vi "Autonomous Independent.vi"() -> ()   [LabVIEW 2015]
doc: "This VI is called when autonomous begins, and will automatically be terminated when autonomous ends. You can carry out timed or sensor driven robot movement independently without needing to return to the caller."
uses:
  Controls/Time.ctl
  Controls/Speed.ctl
  <vilib>/Rock Robotics/WPI/Solenoid/WPI_SolenoidValue.ctl
  <vilib>/Rock Robotics/Network Tables/NT Read String.vi
  <vilib>/Rock Robotics/WPI/Utilities/WPI_GetSetVariantRefNum.vi
  <vilib>/Rock Robotics/Network Tables/NT Write Numeric Array.vi
  <vilib>/Rock Robotics/WPI/Solenoid/WPI_SolenoidSetEnum.vi
  <vilib>/Rock Robotics/Network Tables/NT Write Boolean.vi
  <vilib>/Rock Robotics/Network Tables/NT Read Boolean.vi
panel:
  out "Green":bool
  # "Be sure to right-click and choose Data Operations>>Make Current Value default if you want to save the array values with the VI"
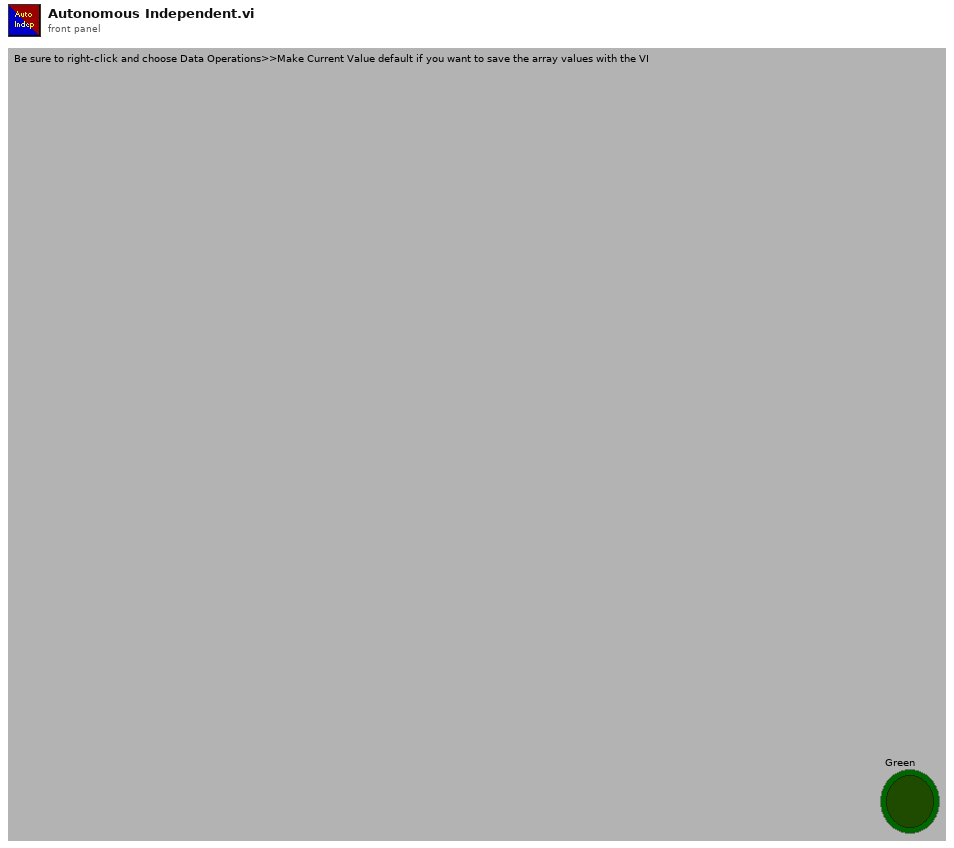
[diagram p1: front panel]
types:
  T1 = typedef "WPI_MotorControlDeviceRef.ctl" = cluster{"DeviceStatus":errorcluster, "Type":T2, "PWM":cluster{"PWM Channel":T3, "DeadBand":T4}, "CAN":cluster{"Device Number":u8, "Control Mode":T5, "Semaphore":T6, "Max Vout":dbl, "TalonSRX Control Mode":T7}, "Invert":bool}
  T2 = typedef "WPI_MotorControlType.ctl" = enum16{"PWM", "CAN", "CANTalonSRX"}
  T3 = typedef "FPGA_DIOPWMChannel.ctl" = enum8{"PWM 0", "PWM 1", "PWM 2", "PWM 3", "PWM 4", "PWM 5", "PWM 6", "PWM 7", "PWM 8", "PWM 9", "PWM MXP 0", "PWM MXP 1", "PWM MXP 2", "PWM MXP 3", "PWM MXP 4", "PWM MXP 5", "PWM MXP 6", "PWM MXP 7", "PWM MXP 8", "PWM MXP 9", "Invalid"}
  T4 = typedef "WPI_PWMDeadband.ctl" = cluster{"Name":string, "maxPositivePwm":i32, "minPositivePwm":i32, "centerPwm":i32, "maxNegativePwm":i32, "minNegativePwm":i32, "angularRange":u16}
  T5 = typedef "WPI_CANJaguar_ControlMode.ctl" = enum8{"Percent VBus", "Current", "Speed", "Position", "Voltage"}
  T6 = typedef "Semaphore RefNum" = refnum<k1>
  T7 = typedef "WPI_CANTalonSRX_APIControlMode.ctl" = enum8{"Percent VBus", "Speed", "Position", "Slave", "Unchanged / Invalid", "Voltage Compensation", "Current", "Motion Profile"}
  T8 = typedef "WPI_JoystickDevRef.ctl" = cluster{"Device":T9}
  T9 = typedef "WPI_JoystickDeviceEnum.ctl" = enum16{"USB 0", "USB 1", "USB 2", "USB 3", "USB 4", "USB 5"}
  T10 = typedef "WPI_RobotDriveDevRef.ctl" = cluster{"DevStatus":errorcluster, "Motors[]":T1[], "Square Inputs":bool, "Max Output":dbl}
  T11 = typedef "Speed.ctl" = dbl
  T12 = typedef "Time.ctl" = dbl
  T13 = typedef "WPI_SolenoidValue.ctl" = enum16{"Off", "On", "Forward", "Reverse"}
  T14 = typedef "WPI_SolenoidDevRef.ctl" = cluster{"DevStatus":errorcluster, "Pneumatics Control Module":u8, "Forward Solenoid Channel":T15, "Reverse Solenoid Channel":T15}
  T15 = typedef "WPI_SolenoidChannel.ctl" = enum8{"Solenoid 0", "Solenoid 1", "Solenoid 2", "Solenoid 3", "Solenoid 4", "Solenoid 5", "Solenoid 6", "Solenoid 7", "Invalid"}
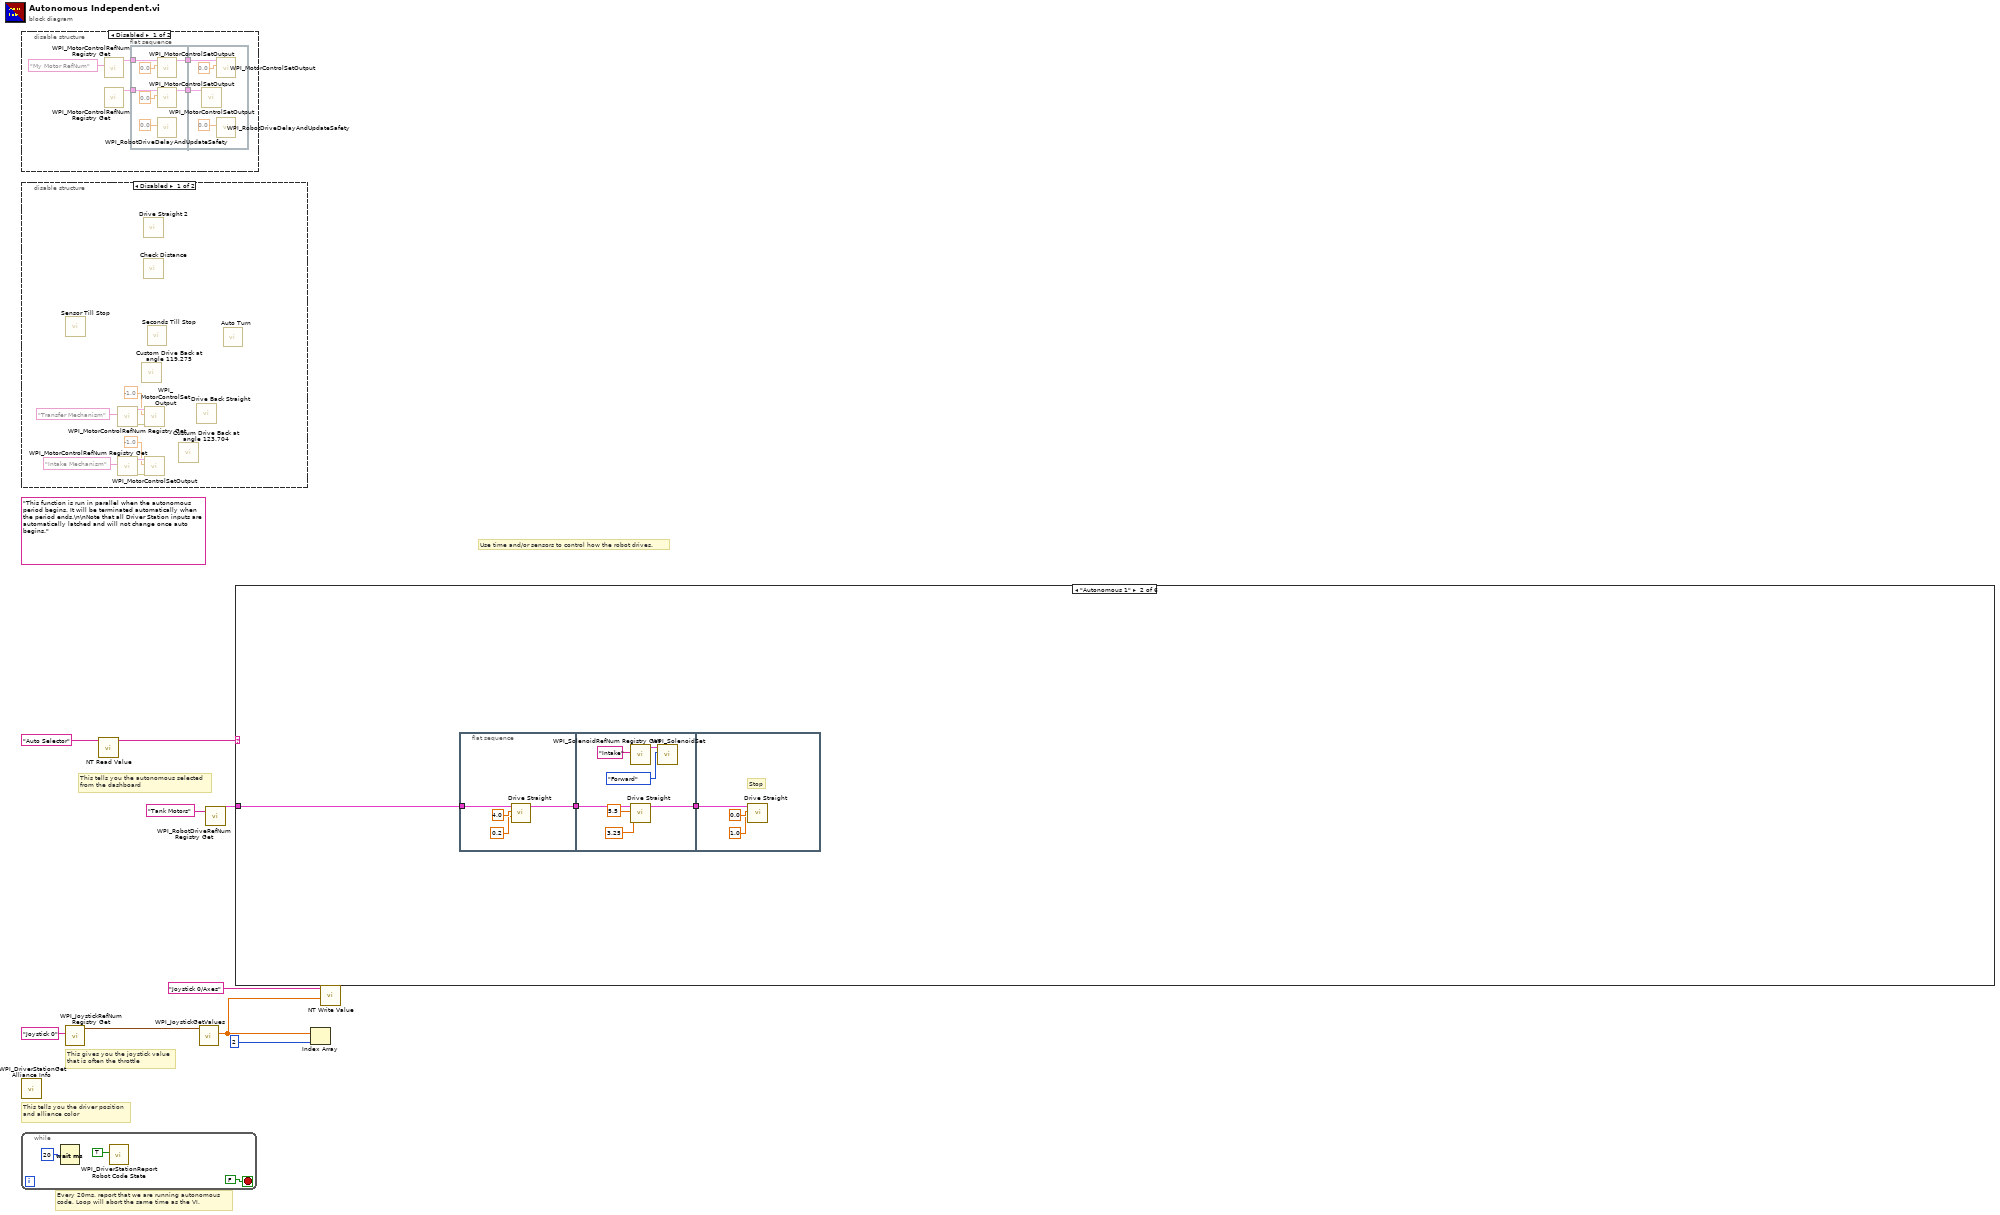
[diagram p0: block diagram]
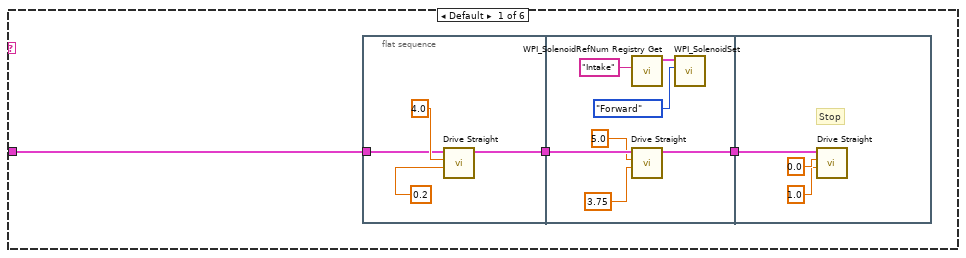
[diagram p4: hidden frame]
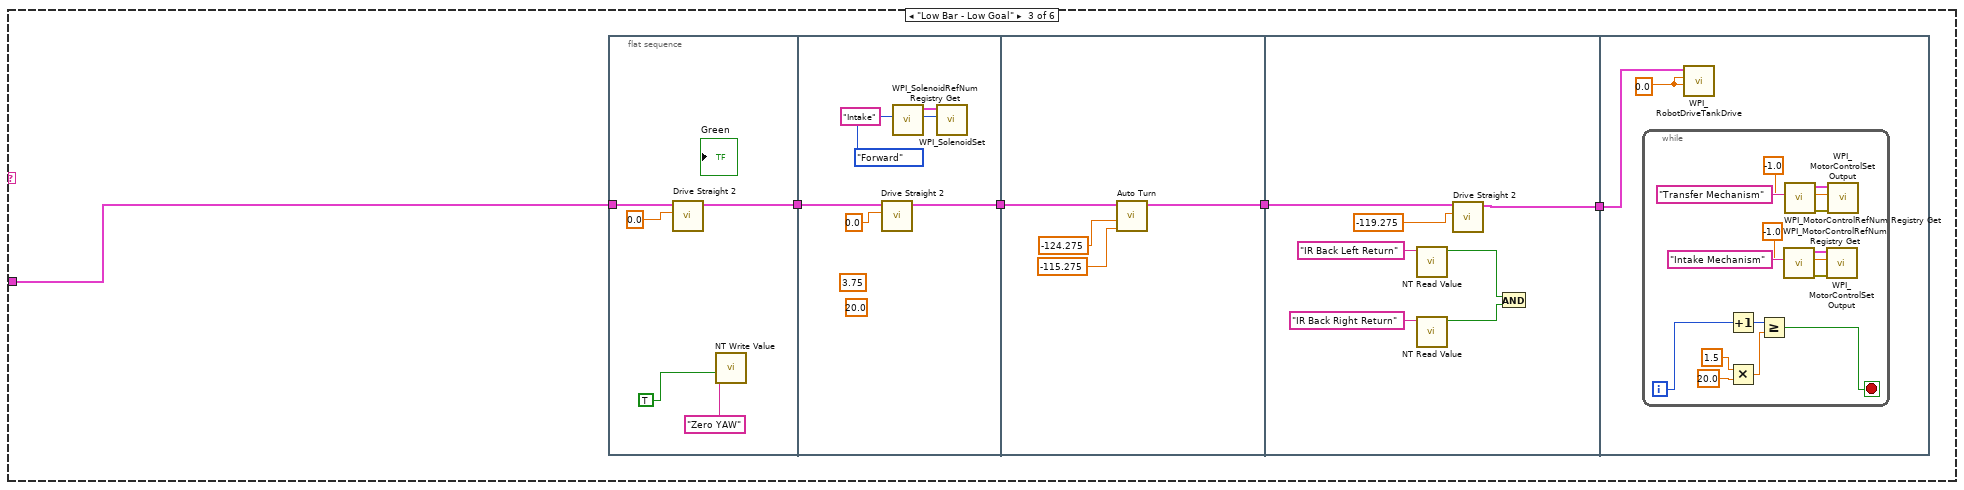
[diagram p5: hidden frame]
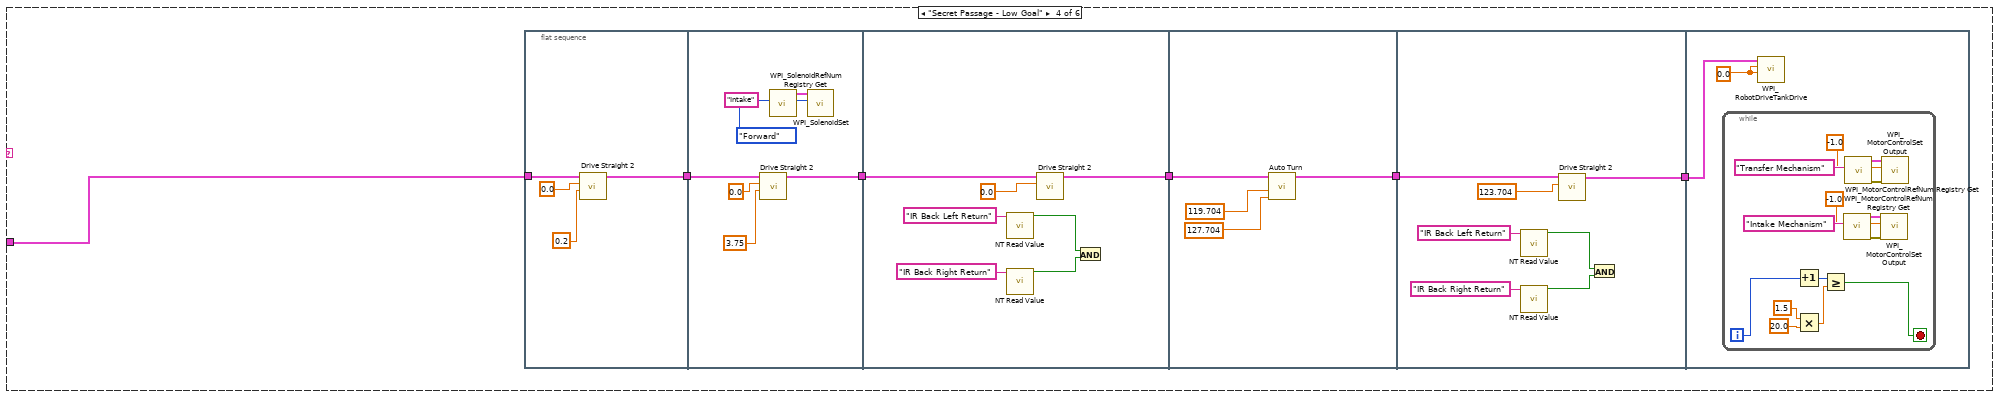
[diagram p6: hidden frame]
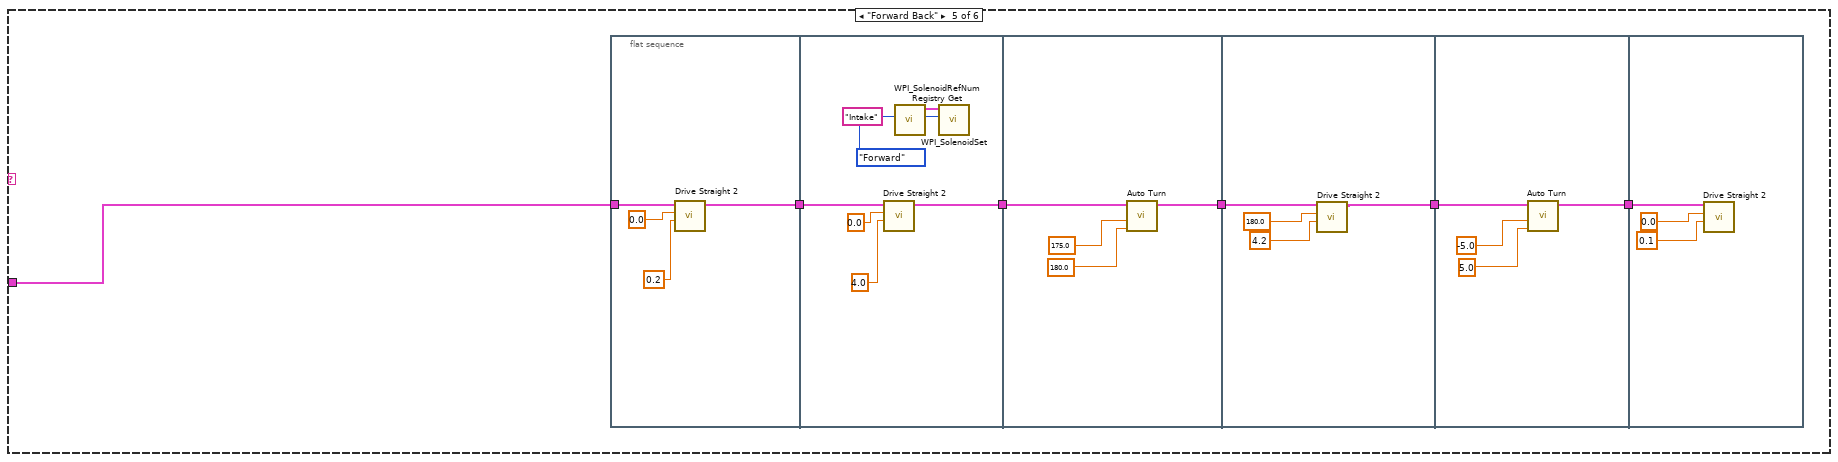
[diagram p7: hidden frame]
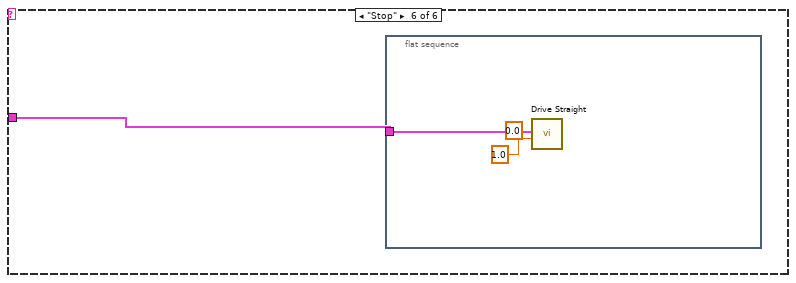
[diagram p8: hidden frame]
diagram:
  (unwired) "This function is run in parallel when the autonomous period begins. It will be terminated automatically when the period ends.\n\nNote that all Driver Station inputs are automatically latched and will not change once auto begins."
  # "This gives you the joystick value\nthat is often the throttle"
  # "This tells you the autonomous selected\nfrom the dashboard"
  # "Every 20ms, report that we are running autonomous\ncode. Loop will abort the same time as the VI."
  # "Use time and/or sensors to control how the robot drives."
  # "This tells you the driver position\nand alliance color"
  n1 = disable-structure shown="Disabled" {
    frame Disabled {
      n2 = call <vilib>:"WPI_MotorControlRefNum Registry Get.vi"("refnum name"="My Motor RefNum") -> ("MotorControlDevRef"=w11:T1)  [unwired: 9 in, 1 out]
      n3 = call <vilib>:"WPI_MotorControlRefNum Registry Get.vi"() -> ("MotorControlDevRef"=w10:T1)  [unwired: 10 in, 1 out]
      n4 = flat-sequence {
        tunnel: w11 -> [w21]
        tunnel: [w18] -> w14
        tunnel: w10 -> [w15]
        tunnel: [w16] -> w13
        tunnel: w14 -> [w23]
        tunnel: w13 -> [w22]
        frame #0 {
          n5 = call <vilib>:"WPI_MotorControlSetOutput.vi"("Output"=0.0, "MotorControlDevRef"=w21) -> ("MotorControlDevRef"=w18:T1)  [unwired: 7 in, 2 out]
          n6 = call <vilib>:"WPI_MotorControlSetOutput.vi"("Output"=0.0, "MotorControlDevRef"=w15) -> ("MotorControlDevRef"=w16:T1)  [unwired: 7 in, 2 out]
          n7 = call <vilib>:"WPI_RobotDriveDelayAndUpdateSafety.vi"("Delay (s)"=0.0) -> ()  [unwired: 9 in, 2 out]
        }
        frame #1 {
          n8 = call <vilib>:"WPI_MotorControlSetOutput.vi"("MotorControlDevRef"=w22) -> ()  [unwired: 8 in, 3 out]
          n9 = call <vilib>:"WPI_MotorControlSetOutput.vi"("Output"=0.0, "MotorControlDevRef"=w23) -> ()  [unwired: 7 in, 3 out]
          n10 = call <vilib>:"WPI_RobotDriveDelayAndUpdateSafety.vi"("Delay (s)"=0.0) -> ()  [unwired: 9 in, 2 out]
        }
      }
    }
    frame Enabled {
    }
  }
  n11 = disable-structure shown="Disabled" {
    frame Disabled {
      n12 = call "Sensor Till Stop.vi"() -> ()  [unwired: 11 in, 1 out]
      n13 = call <vilib>:"WPI_MotorControlRefNum Registry Get.vi"("refnum name"="Transfer Mechanism") -> ("error out"=w30:errorcluster, "MotorControlDevRef"=w28:T1)  [unwired: 9 in]
      n14 = call <vilib>:"WPI_MotorControlRefNum Registry Get.vi"("refnum name"="Intake Mechanism") -> ("error out"=w33:errorcluster, "MotorControlDevRef"=w32:T1)  [unwired: 9 in]
      n15 = call "Custom Drive Back at angle 119.275.vi"() -> ()  [unwired: 10 in, 2 out]
      n16 = call "Drive Straight 2.vi"() -> ()  [unwired: 11 in, 1 out]
      n17 = call "Check Distance.vi"() -> ()  [unwired: 11 in, 1 out]
      n18 = call <vilib>:"WPI_MotorControlSetOutput.vi"("error in (no error)"=w30, "Output"=-1.0, "MotorControlDevRef"=w28) -> ()  [unwired: 6 in, 3 out]
      n19 = call <vilib>:"WPI_MotorControlSetOutput.vi"("error in (no error)"=w33, "Output"=-1.0, "MotorControlDevRef"=w32) -> ()  [unwired: 6 in, 3 out]
      n20 = call "Seconds Till Stop.vi"() -> ()  [unwired: 11 in, 1 out]
      n21 = call "Custum Drive Back at angle 123.704.vi"() -> ()  [unwired: 10 in, 2 out]
      n22 = call "Drive Back Straight.vi"() -> ()  [unwired: 10 in, 2 out]
      n23 = call "Auto Turn.vi"() -> ()  [unwired: 11 in, 1 out]
    }
    frame Enabled {
    }
  }
  n24 = call <vilib>:"WPI_DriverStationGet Alliance Info.vi"() -> ()  [unwired: 12 out]
  n25 = while {
    stop <- FALSE stop-if-true
    n26 = Wait (ms)(milliseconds to wait=u32 20) -> ()  [unwired: 1 out]
    n27 = call <vilib>:"WPI_DriverStationReport Robot Code State.vi"("Autonomous"=TRUE) -> ()  [unwired: 10 in, 1 out]
  }
  n28 = call <vilib>:"WPI_JoystickRefNum Registry Get.vi"("refnum name"="Joystick 0") -> ("JoystickDevRef"=w6:T8)  [unwired: 1 in, 9 out]
  n29 = call-poly <vilib>:"NT Read Value.vi"("Name"="Auto Selector") -> ("String"=w8:string)  [unwired: 9 in, 1 out]
  n30 = call <vilib>:"WPI_JoystickGetValues.vi"("JoystickDevRef"=w6) -> ("Axes"=w4:dbl[])  [unwired: 6 in, 4 out]
  n31 = call <vilib>:"WPI_RobotDriveRefNum Registry Get.vi"("refnum name"="Tank Motors") -> ("RobotDriveDevRef"=w1:T10)  [unwired: 9 in, 1 out]
  n32 = case shown="\"Autonomous 1\"" w8 {
    tunnel: w1 -> [w37 w54 w75 w119 w170 w197]
    frame Default {
      n33 = flat-sequence {
        tunnel: [w41] -> w39
        tunnel: w37 -> [w40]
        tunnel: w39 -> [w47]
        tunnel: [w44] -> w38
        tunnel: w38 -> [w53]
        frame #0 {
          n34 = call "Drive Straight.vi"("Time"=T12 0.2, "Speed"=T11 4.0, "RobotDriveDevRef"=w40) -> ("RobotDriveDevRef 2"=w41:T10)  [unwired: 8 in]
        }
        frame #1 {
          n35 = call <vilib>:"WPI_SolenoidRefNum Registry Get.vi"("refnum name"="Intake") -> ("SolenoidDevRef"=w49:T14)  [unwired: 9 in, 1 out]
          n36 = call "Drive Straight.vi"("Time"=T12 3.75, "Speed"=T11 5.0, "RobotDriveDevRef"=w47) -> ("RobotDriveDevRef 2"=w44:T10)  [unwired: 8 in]
          n37 = call-poly <vilib>:"WPI_SolenoidSet.vi"("Value"=WPI_SolenoidValue."Forward", "SolenoidDevRef"=w49) -> ()  [unwired: 1 in, 9 out]
        }
        frame #2 {
          # "Stop"
          n38 = call "Drive Straight.vi"("Time"=T12 1.0, "Speed"=T11 0.0, "RobotDriveDevRef"=w53) -> ()  [unwired: 8 in, 1 out]
        }
      }
    }
    frame "Autonomous 1" {
      n39 = flat-sequence {
        tunnel: [w58] -> w56
        tunnel: w54 -> [w57]
        tunnel: w56 -> [w67]
        tunnel: [w65] -> w55
        tunnel: w55 -> [w70]
        frame #0 {
          n40 = call "Drive Straight.vi"("Time"=T12 0.2, "Speed"=T11 4.0, "RobotDriveDevRef"=w57) -> ("RobotDriveDevRef 2"=w58:T10)  [unwired: 8 in]
        }
        frame #1 {
          n41 = call <vilib>:"WPI_SolenoidRefNum Registry Get.vi"("refnum name"="Intake") -> ("SolenoidDevRef"=w63:T14)  [unwired: 9 in, 1 out]
          n42 = call "Drive Straight.vi"("Time"=T12 3.25, "Speed"=T11 5.5, "RobotDriveDevRef"=w67) -> ("RobotDriveDevRef 2"=w65:T10)  [unwired: 8 in]
          n43 = call-poly <vilib>:"WPI_SolenoidSet.vi"("Value"=WPI_SolenoidValue."Forward", "SolenoidDevRef"=w63) -> ()  [unwired: 1 in, 9 out]
        }
        frame #2 {
          # "Stop"
          n44 = call "Drive Straight.vi"("Time"=T12 1.0, "Speed"=T11 0.0, "RobotDriveDevRef"=w70) -> ()  [unwired: 8 in, 1 out]
        }
      }
    }
    frame "Low Bar - Low Goal" {
      n45 = flat-sequence {
        tunnel: [w78] -> w73
        tunnel: w75 -> [w80]
        tunnel: w73 -> [w82]
        tunnel: [w81] -> w71
        tunnel: [w90] -> w74
        tunnel: w71 -> [w87]
        tunnel: w74 -> [w92]
        tunnel: [w91] -> w72
        tunnel: w72 -> [w99]
        frame #0 {
          n46 = call "Drive Straight 2.vi"("Angle"=0.0, "RobotDriveDevRef in"=w80) -> ("RobotDriveDevRef out"=w78:T10)  [unwired: 9 in]
          n47 = call-poly <vilib>:"NT Write Value.vi"("Boolean"=TRUE, "Name"="Zero YAW") -> ()  [unwired: 9 in, 1 out]
        }
        frame #1 {
          (unwired) 20.0 ("y")
          (unwired) 3.75 ("Time")
          n48 = call "Drive Straight 2.vi"("Angle"=0.0, "RobotDriveDevRef in"=w82) -> ("RobotDriveDevRef out"=w81:T10)  [unwired: 9 in]
          n49 = call <vilib>:"WPI_SolenoidRefNum Registry Get.vi"("refnum name"="Intake") -> ("SolenoidDevRef"=w85:T14)  [unwired: 9 in, 1 out]
          n50 = call-poly <vilib>:"WPI_SolenoidSet.vi"("Value"=WPI_SolenoidValue."Forward", "SolenoidDevRef"=w85) -> ()  [unwired: 1 in, 9 out]
        }
        frame #2 {
          n51 = call "Auto Turn.vi"("upper limit"=-115.275 ("lower limit"), "lower limit"=-124.275 ("upper limit"), "RobotDriveDevRef"=w87) -> ("RobotDriveDevRef out"=w90:T10)  [unwired: 8 in]
        }
        frame #3 {
          n52 = call-poly <vilib>:"NT Read Value.vi"("Name"="IR Back Left Return") -> ("Boolean"=w94:bool)  [unwired: 9 in, 1 out]
          n53 = call-poly <vilib>:"NT Read Value.vi"("Name"="IR Back Right Return") -> ("Boolean"=w95:bool)  [unwired: 9 in, 1 out]
          n54 = call "Drive Straight 2.vi"("Angle"=-119.275, "RobotDriveDevRef in"=w92) -> ("RobotDriveDevRef out"=w91:T10)  [unwired: 9 in]
          n55 = And(x=w94, y=w95) -> ()  [unwired: 1 out]
        }
        frame #4 {
          w98 = 0.0 ("Angle")
          n56 = while {
            i -> [w101]
            stop <- w100 stop-if-true
            n57 = Increment(x=w101) -> (x+1=w103:i32)
            n58 = Multiply(x=1.5 ("Time"), y=20.0) -> (x*y=w104:dbl)
            n59 = Greater Or Equal?(x=w103, y=w104) -> (x >= y?=w100:bool)
            n60 = call <vilib>:"WPI_MotorControlRefNum Registry Get.vi"("refnum name"="Intake Mechanism") -> ("error out"=w113:errorcluster, "MotorControlDevRef"=w112:T1)  [unwired: 9 in]
            n61 = call <vilib>:"WPI_MotorControlRefNum Registry Get.vi"("refnum name"="Transfer Mechanism") -> ("error out"=w110:errorcluster, "MotorControlDevRef"=w108:T1)  [unwired: 9 in]
            n62 = call <vilib>:"WPI_MotorControlSetOutput.vi"("error in (no error)"=w113, "Output"=-1.0, "MotorControlDevRef"=w112) -> ()  [unwired: 6 in, 3 out]
            n63 = call <vilib>:"WPI_MotorControlSetOutput.vi"("error in (no error)"=w110, "Output"=-1.0, "MotorControlDevRef"=w108) -> ()  [unwired: 6 in, 3 out]
          }
          n64 = call <vilib>:"WPI_RobotDriveTankDrive.vi"("Right axis value"=w98, "Left axis value"=w98, "RobotDriveDevRef"=w99) -> ()  [unwired: 6 in, 3 out]
        }
      }
    }
    frame "Secret Passage - Low Goal" {
      n65 = flat-sequence {
        tunnel: [w121] -> w115
        tunnel: w119 -> [w123]
        tunnel: [w127] -> w118
        tunnel: w115 -> [w125]
        tunnel: w118 -> [w137]
        tunnel: [w135] -> w117
        tunnel: w117 -> [w141]
        tunnel: [w140] -> w116
        tunnel: w116 -> [w143]
        tunnel: [w142] -> w114
        tunnel: w114 -> [w150]
        frame #0 {
          n66 = call "Drive Straight 2.vi"("Time"=0.2, "Angle"=0.0, "RobotDriveDevRef in"=w123) -> ("RobotDriveDevRef out"=w121:T10)  [unwired: 8 in]
        }
        frame #1 {
          n67 = call "Drive Straight 2.vi"("Time"=3.75, "Angle"=0.0, "RobotDriveDevRef in"=w125) -> ("RobotDriveDevRef out"=w127:T10)  [unwired: 8 in]
          n68 = call <vilib>:"WPI_SolenoidRefNum Registry Get.vi"("refnum name"="Intake") -> ("SolenoidDevRef"=w129:T14)  [unwired: 9 in, 1 out]
          n69 = call-poly <vilib>:"WPI_SolenoidSet.vi"("Value"=WPI_SolenoidValue."Forward", "SolenoidDevRef"=w129) -> ()  [unwired: 1 in, 9 out]
        }
        frame #2 {
          n70 = call-poly <vilib>:"NT Read Value.vi"("Name"="IR Back Left Return") -> ("Boolean"=w134:bool)  [unwired: 9 in, 1 out]
          n71 = call-poly <vilib>:"NT Read Value.vi"("Name"="IR Back Right Return") -> ("Boolean"=w133:bool)  [unwired: 9 in, 1 out]
          n72 = call "Drive Straight 2.vi"("Angle"=0.0, "RobotDriveDevRef in"=w137) -> ("RobotDriveDevRef out"=w135:T10)  [unwired: 9 in]
          n73 = And(x=w134, y=w133) -> ()  [unwired: 1 out]
        }
        frame #3 {
          n74 = call "Auto Turn.vi"("upper limit"=127.704, "lower limit"=119.704, "RobotDriveDevRef"=w141) -> ("RobotDriveDevRef out"=w140:T10)  [unwired: 8 in]
        }
        frame #4 {
          n75 = call-poly <vilib>:"NT Read Value.vi"("Name"="IR Back Left Return") -> ("Boolean"=w145:bool)  [unwired: 9 in, 1 out]
          n76 = call-poly <vilib>:"NT Read Value.vi"("Name"="IR Back Right Return") -> ("Boolean"=w146:bool)  [unwired: 9 in, 1 out]
          n77 = call "Drive Straight 2.vi"("Angle"=123.704, "RobotDriveDevRef in"=w143) -> ("RobotDriveDevRef out"=w142:T10)  [unwired: 9 in]
          n78 = And(x=w145, y=w146) -> ()  [unwired: 1 out]
        }
        frame #5 {
          w149 = 0.0 ("Angle")
          n79 = while {
            i -> [w152]
            stop <- w151 stop-if-true
            n80 = Increment(x=w152) -> (x+1=w154:i32)
            n81 = Multiply(x=1.5 ("Time"), y=20.0) -> (x*y=w155:dbl)
            n82 = Greater Or Equal?(x=w154, y=w155) -> (x >= y?=w151:bool)
            n83 = call <vilib>:"WPI_MotorControlRefNum Registry Get.vi"("refnum name"="Intake Mechanism") -> ("error out"=w164:errorcluster, "MotorControlDevRef"=w163:T1)  [unwired: 9 in]
            n84 = call <vilib>:"WPI_MotorControlRefNum Registry Get.vi"("refnum name"="Transfer Mechanism") -> ("error out"=w161:errorcluster, "MotorControlDevRef"=w159:T1)  [unwired: 9 in]
            n85 = call <vilib>:"WPI_MotorControlSetOutput.vi"("error in (no error)"=w164, "Output"=-1.0, "MotorControlDevRef"=w163) -> ()  [unwired: 6 in, 3 out]
            n86 = call <vilib>:"WPI_MotorControlSetOutput.vi"("error in (no error)"=w161, "Output"=-1.0, "MotorControlDevRef"=w159) -> ()  [unwired: 6 in, 3 out]
          }
          n87 = call <vilib>:"WPI_RobotDriveTankDrive.vi"("Right axis value"=w149, "Left axis value"=w149, "RobotDriveDevRef"=w150) -> ()  [unwired: 6 in, 3 out]
        }
      }
    }
    frame "Forward Back" {
      n88 = flat-sequence {
        tunnel: [w172] -> w167
        tunnel: w170 -> [w174]
        tunnel: [w178] -> w169
        tunnel: w167 -> [w176]
        tunnel: [w185] -> w168
        tunnel: w169 -> [w182]
        tunnel: w168 -> [w188]
        tunnel: [w186] -> w166
        tunnel: w166 -> [w191]
        tunnel: [w190] -> w165
        tunnel: w165 -> [w194]
        frame #0 {
          n89 = call "Drive Straight 2.vi"("Time"=0.2, "Angle"=0.0, "RobotDriveDevRef in"=w174) -> ("RobotDriveDevRef out"=w172:T10)  [unwired: 8 in]
        }
        frame #1 {
          n90 = call "Drive Straight 2.vi"("Time"=4.0, "Angle"=0.0, "RobotDriveDevRef in"=w176) -> ("RobotDriveDevRef out"=w178:T10)  [unwired: 8 in]
          n91 = call <vilib>:"WPI_SolenoidRefNum Registry Get.vi"("refnum name"="Intake") -> ("SolenoidDevRef"=w180:T14)  [unwired: 9 in, 1 out]
          n92 = call-poly <vilib>:"WPI_SolenoidSet.vi"("Value"=WPI_SolenoidValue."Forward", "SolenoidDevRef"=w180) -> ()  [unwired: 1 in, 9 out]
        }
        frame #2 {
          n93 = call "Auto Turn.vi"("upper limit"=180.0, "lower limit"=175.0, "RobotDriveDevRef"=w182) -> ("RobotDriveDevRef out"=w185:T10)  [unwired: 8 in]
        }
        frame #3 {
          n94 = call "Drive Straight 2.vi"("Time"=4.2 ("Angle"), "Angle"=180.0, "RobotDriveDevRef in"=w188) -> ("RobotDriveDevRef out"=w186:T10)  [unwired: 8 in]
        }
        frame #4 {
          n95 = call "Auto Turn.vi"("upper limit"=5.0, "lower limit"=-5.0, "RobotDriveDevRef"=w191) -> ("RobotDriveDevRef out"=w190:T10)  [unwired: 8 in]
        }
        frame #5 {
          n96 = call "Drive Straight 2.vi"("Time"=0.1 ("Angle"), "Angle"=0.0, "RobotDriveDevRef in"=w194) -> ()  [unwired: 8 in, 1 out]
        }
      }
    }
    frame "Stop" {
      n97 = flat-sequence {
        tunnel: w197 -> [w200]
        frame #0 {
          n98 = call "Drive Straight.vi"("Time"=T12 1.0, "Speed"=T11 0.0, "RobotDriveDevRef"=w200) -> ()  [unwired: 8 in, 1 out]
        }
      }
    }
  }
  n99 = Index Array(array=w4, index=2) -> ()  [unwired: 1 out]
  n100 = call-poly <vilib>:"NT Write Value.vi"("Numeric Array"=w4, "Name"="Joystick 0/Axes") -> ()  [unwired: 9 in, 1 out]
